vi "Write Position.vi"(8 "error in (no error)":errorcluster, 9 "Position":T1, 11 "Char LCD I in":refnum<class "Char LCD.lvclass">) -> (0 "error out":errorcluster, 3 "Char LCD I out":refnum<class "Char LCD.lvclass">)   [LabVIEW 2020, in "CTI-Peripheral.lvlib" / "Char LCD.lvclass"]
uses:
  Char LCD.lvclass
  Position.ctl
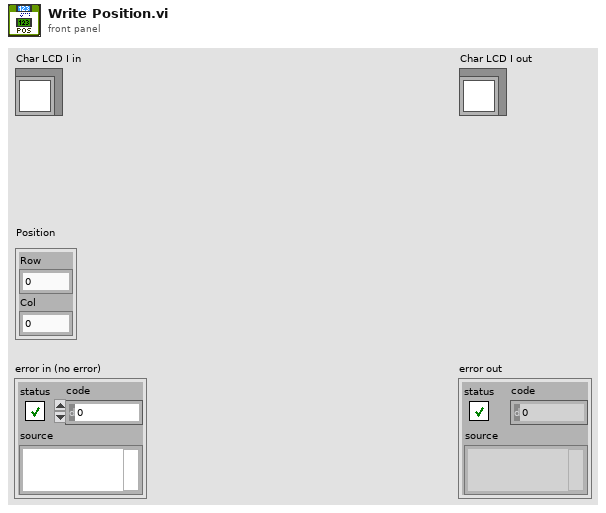
[diagram p1: front panel]
types:
  T1 = typedef "CTI-Peripheral.lvlib/Char LCD.lvclass/Position.ctl" = cluster{"Row":u8, "Col":u8}
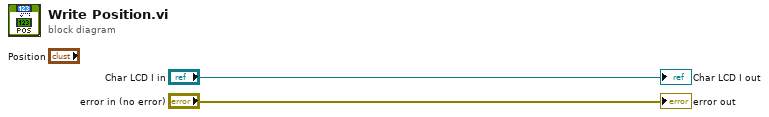
[diagram p0: block diagram]
diagram:
  "error out" <- "error in (no error)"
  "Char LCD I out" <- "Char LCD I in"
